vi "Get COM semaphore.vi"(8 "error in (no error)":errorcluster, 10 "create if not found (T)":bool, 11 "VISA resource in":refnum<visa-resource-name>) -> (0 "error out":errorcluster, 2 "semaphore":T1, 3 "VISA resource out":refnum<visa-resource-name>)   [LabVIEW 2020, in "Global FIA milliGAT.lvlib"]
uses:
  <instrlib>/RxnRover/Global FIA milliGAT 3.14/Global FIA milliGAT.lvlib
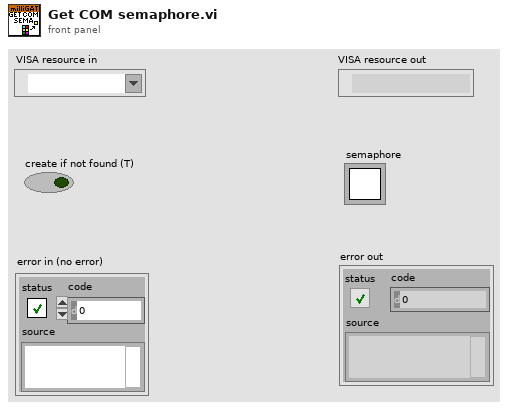
[diagram p1: front panel]
types:
  T1 = typedef "Semaphore RefNum" = refnum<k1>
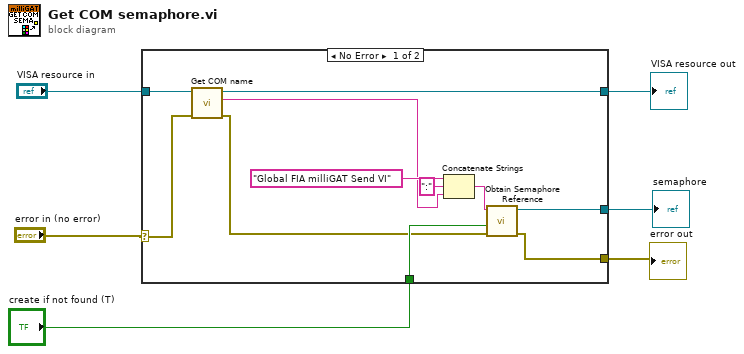
[diagram p0: block diagram]
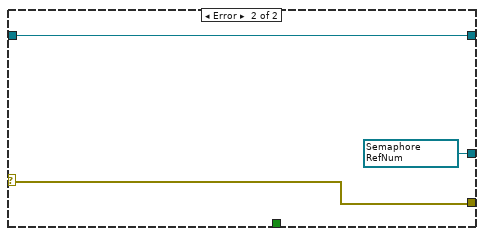
[diagram p2: hidden frame]
diagram:
  n1 = case shown="No Error" "error in (no error)" {
    selector: "error in (no error)" -> [w15 w19]
    tunnel: "VISA resource in" -> [w17 w20]
    tunnel: [w16 w20] -> w5
    tunnel: "create if not found (T)" -> [w14 _]
    tunnel: [w9 w18] -> w2
    tunnel: [w7 w19] -> w1
    frame No Error {
      n2 = call <instrlib>:"Get COM name.vi"("error in (no error)"=w15, "VISA resource in"=w17) -> ("error IO"=w8:errorcluster, "COM name"=w11:string, "VISA resource out"=w16:refnum<visa-resource-name>)  [unwired: 7 in]
      n3 = Concatenate Strings("Global FIA milliGAT Send VI" ("name (unnamed)"), ":" ("string"), w11) -> (w10:string)
      n4 = call <vilib>:"Obtain Semaphore Reference.vi"("error in (no error)"=w8, "create if not found (T)"=w14, "name (unnamed)"=w10) -> ("error out"=w7:errorcluster, "semaphore"=w9:T1)  [unwired: 2 in, 1 out]
    }
    frame Error {
      w18 = T1 refnum items=["semaphore"] ("semaphore")
    }
  }
  "VISA resource out" <- w5
  "semaphore" <- w2
  "error out" <- w1
